vi "Write Binary Config.vi"(4 "Include Class Name":bool, 6 "byte order (0:big-endian, network order)":T1(ring), 8 "error in (no error)":errorcluster, 11 "AbsFunc_One Term_DBL in":refnum<class "AbsFunc_One Term_Time.lvclass">) -> (0 "error out":errorcluster, 2 "Binary":string, 3 "AbsFunc_One Term_DBL out":refnum<class "AbsFunc_One Term_Time.lvclass">)   [LabVIEW 2021, in "AbsFunc_One Term_Time.lvclass"]
uses:
  AbsFunc_One Term_Time.lvclass
  AbsFunc_One Term_Time.lvclass/AbsFunc_One Term_Time.ctl
  Abs_Types/Time/Abs_Time.lvclass
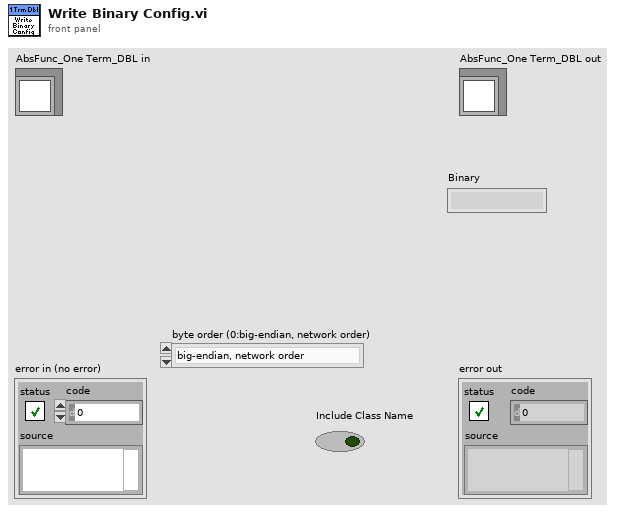
[diagram p1: front panel]
types:
  T1 = enum16{"big-endian, network order", "native, host order", "little-endian"}
  T2 = typedef "AbsFunc_One Term_Time.lvclass/Abstract Type.ctl" = refnum<class "Abs_Time.lvclass">
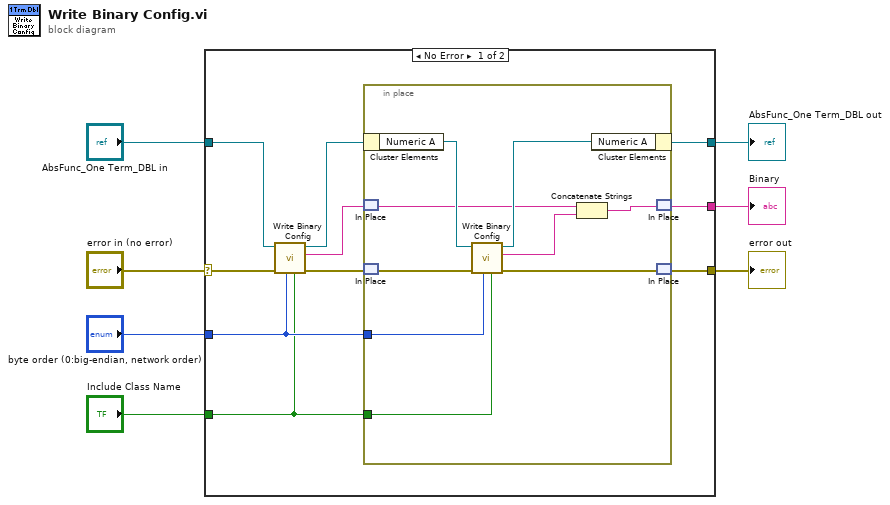
[diagram p0: block diagram]
diagram:
  n1 = case shown="No Error" "error in (no error)" {
    selector: "error in (no error)" -> [w17 w27]
    tunnel: "AbsFunc_One Term_DBL in" -> [w16 w28]
    tunnel: [w12 _] -> w5
    tunnel: "byte order (0:big-endian, network order)" -> [w11 _]
    tunnel: "Include Class Name" -> [w10 _]
    tunnel: [w9 w27] -> w6
    tunnel: [w8 w28] -> w4
    frame No Error {
      n2 = call-parent "Write Binary Config.vi"("Include Class Name"=w10, "byte order (0:big-endian, network order)"=w11, "error in (no error)"=w17, "Abs_Type in"=w16) -> ("error out"=w14:errorcluster, "Binary"=w13:string, "Abs_Type out"=w15:refnum<class "AbsFunc_One Term_Time.lvclass">)  [unwired: 5 in]
      n3 = in-place {
        in-place-border: w11 -> [w21]
        in-place-border: w10 -> [w23]
        n4 = in-place-cluster #1(w15) -> ("Numeric A"=w24:T2)
        n5 = in-place-match #2(w13) -> (w20:string)
        n6 = in-place-match #3(w14) -> (w26:errorcluster)
        n7 = call-dynamic "Write Binary Config.vi"("Include Class Name"=w23, "byte order (0:big-endian, network order)"=w21, "error in (no error)"=w26, "Abs_Type in"=w24) -> ("error out"=w22:errorcluster, "Binary"=w19:string, "Abs_Type out"=w25:T2)  [unwired: 5 in]
        n8 = Concatenate Strings(w20, w19) -> (w18:string)
        n9 = in-place-cluster #1("Numeric A"=w25) -> (w8:refnum<class "AbsFunc_One Term_Time.lvclass">)
        n10 = in-place-match #2(w18) -> (w12:string)
        n11 = in-place-match #3(w22) -> (w9:errorcluster)
      }
    }
    frame Error {
    }
  }
  "error out" <- w6
  "AbsFunc_One Term_DBL out" <- w4
  "Binary" <- w5
